vi "Alternating LEDS.vi"() -> ()   [LabVIEW 2017]
panel:
  out "Led B":bool
  out "Led A":bool
  in  "stop":bool
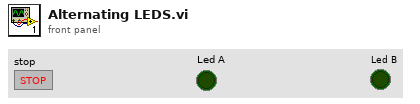
[diagram p1: front panel]
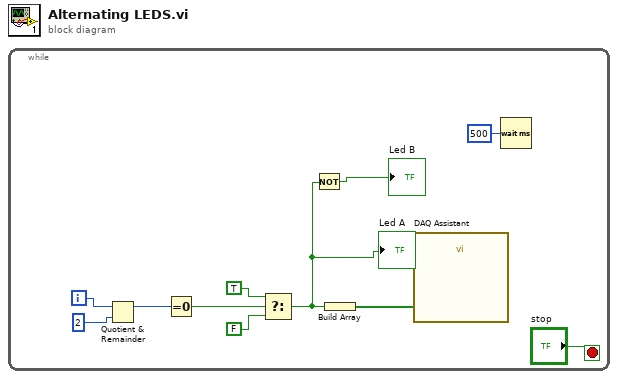
[diagram p0: block diagram]
diagram:
  n1 = while {
    i -> [w10]
    stop <- "stop" stop-if-true
    n2 = Quotient & Remainder(x=w10, y=2) -> (x-y*floor(x/y)=w7:i32)  [unwired: 1 out]
    n3 = Equal To 0?(x=w7) -> (x = 0?=w6:bool)
    n4 = Select(t=TRUE, s=w6, f=FALSE) -> (s? t:f=w2:bool)
    "Led A" <- w2
    n5 = Not(x=w2) -> (.not. x?=→"Led B":bool)
    n6 = Build Array(w2) -> (w3:bool[])
    n7 = call "DAQ Assistant"("data"=w3) -> ()  [unwired: 17 in, 2 out]
    n8 = Wait (ms)(milliseconds to wait=u32 500) -> ()  [unwired: 1 out]
  }
